vi "retrieveTCPSettings.vi"(8 "error in (no error)":errorcluster, 11 "ConfigurationFileReader in":refnum<class "ConfigurationFileReader.lvclass">) -> (0 "error out":errorcluster, 2 "TCPConfiguration":T1={"IP"="127.0.0.1", "port_low"=50000, "port_up"=50000, "connection_timeout "=10, "reading_timeout"=10, "writing_timeout"=10}, 3 "ConfigurationFileReader out":refnum<class "ConfigurationFileReader.lvclass">)   [LabVIEW 2016, in "Settings.lvlib" / "ConfigurationFileReader.lvclass"]
uses:
  ConfigurationFileReader.lvclass
  ConfigurationTypedefs/Base/TCPConfiguration.ctl
  ConfigurationTypedefs/ConfigurationTypedefs.lvlib
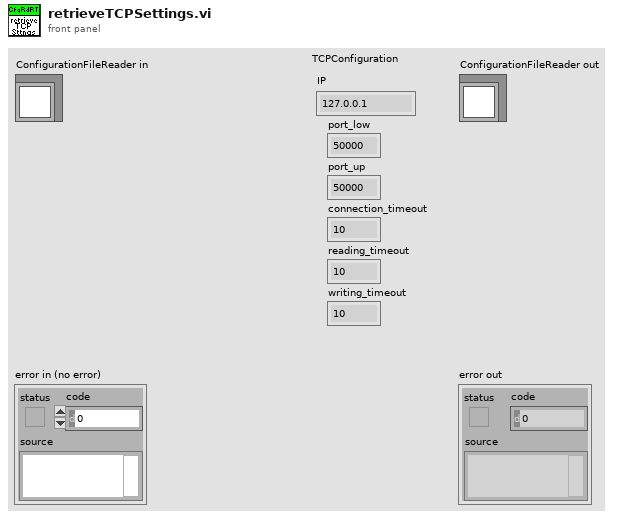
[diagram p1: front panel]
types:
  T1 = typedef "Settings.lvlib/ConfigurationTypedefs.lvlib/TCPConfiguration.ctl" = cluster{"IP":string, "port_low":u16, "port_up":u16, "connection_timeout ":i32, "reading_timeout":i32, "writing_timeout":i32}
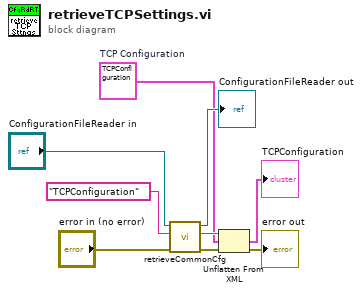
[diagram p0: block diagram]
diagram:
  w1 = T1 {"IP"="127.0.0.1", "port_low"=50000, "port_up"=50000, "connection_timeout "=10, "reading_timeout"=10, "writing_timeout"=10}  # TCP Configuration
  n1 = call "retrieveCommonCfg.vi"("error in (no error)"="error in (no error)", "dataName"="TCPConfiguration", "ConfigurationFileReader in"="ConfigurationFileReader in") -> ("error out"=w7:errorcluster, "dataValueFromFile"=w8:string, "ConfigurationFileReader out"=→"ConfigurationFileReader out":refnum<class "ConfigurationFileReader.lvclass">)  [unwired: 6 in]
  n2 = Unflatten From XML(xml string=w8, type=w1, error in (no error)=w7) -> (value=→"TCPConfiguration":T1, error out=→"error out":errorcluster)
